vi "Decimate 1D by Min-Max Algorythm.vi"(4 "Width":i32, 6 "Packet sizes":i32[](array[numeric]), 8 "error in (no error)":errorcluster, 9 "Min Index":i32, 10 "Max Index":i32, 11 "Data To Decimate":dbl[](array[numeric])) -> (0 "error out":errorcluster, 3 "Decimated Data":dbl[](array[numeric]))   [LabVIEW 2022 SP3, in "Decimation.lvlib"]
uses:
  Decimation.lvlib
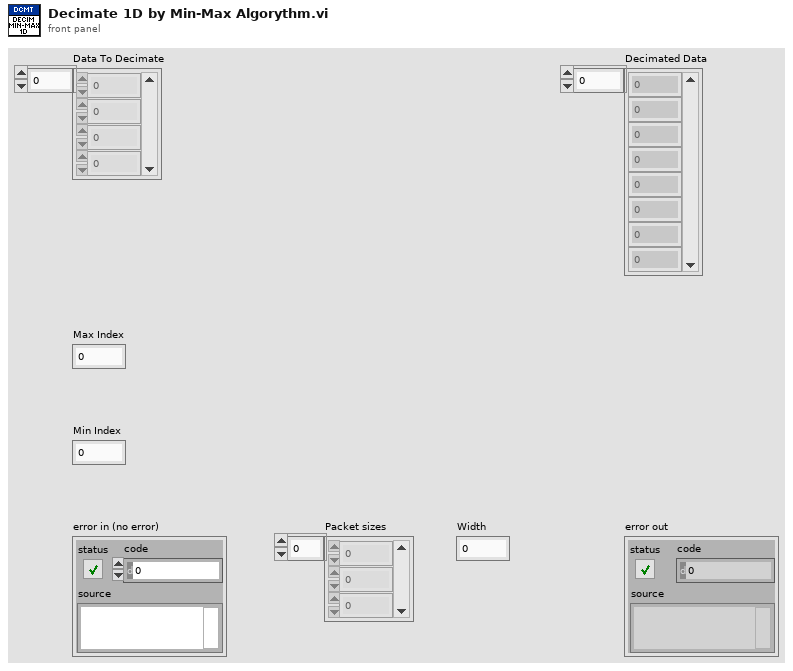
[diagram p1: front panel]
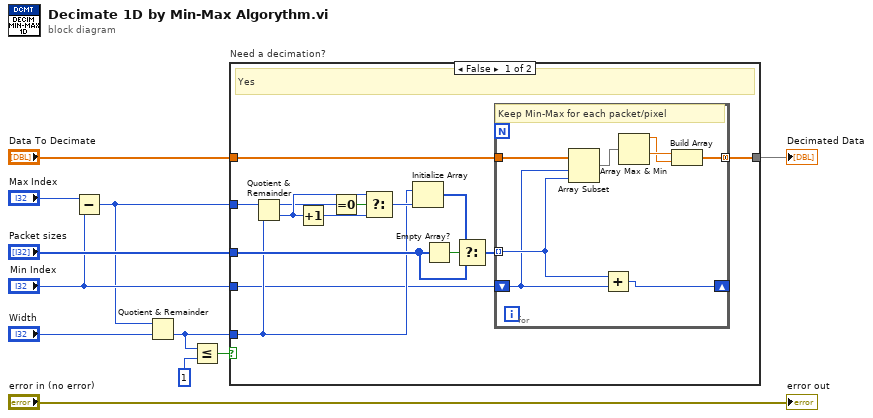
[diagram p0: block diagram]
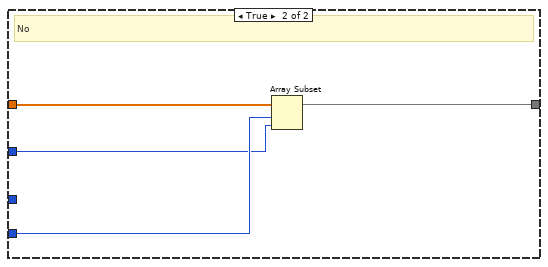
[diagram p2: hidden frame]
diagram:
  n1 = Subtract(x="Max Index", y="Min Index") -> (x-y=w1:i32)
  n2 = Quotient & Remainder(x=w1, y="Width") -> (floor(x/y)=w2:i32)  [unwired: 1 out]
  n3 = Less Or Equal?(x=w2, y=u32 1) -> (x <= y?=w6:bool)
  n4 = case "Need a decimation?" shown="False" w6 {
    tunnel: "Packet sizes" -> [w22 _]
    tunnel: "Data To Decimate" -> [w25 w37]
    tunnel: [w24 w36] -> w11
    tunnel: "Min Index" -> [w12 w35]
    tunnel: w2 -> [w13 _]
    tunnel: w1 -> [w20 w34]
    frame False {
      # "Yes"
      n5 = Quotient & Remainder(x=w20, y=w13) -> (x-y*floor(x/y)=w16:i32, floor(x/y)=w17:i32)
      n6 = Increment(x=w17) -> (x+1=w18:i32)
      n7 = Equal To 0?(x=w16) -> (x = 0?=w19:bool)
      n8 = Select(t=w17, s=w19, f=w18) -> (s? t:f=w14:i32)
      n9 = Initialize Array(w13, w14) -> (w15:i32[])
      n10 = Empty Array?(array=w22) -> (empty?=w23:bool)
      n11 = Select(t=w15, s=w23, f=w22) -> (s? t:f=w21:i32[])
      n12 = for {
        tunnel: [w32] -> w24 mode=concatenating
        tunnel: w21 -> [w28] mode=indexing
        shift-right: [w26] -> _
        shift-left: w12 -> [w27]
        tunnel: w25 -> [w33]
        # "Keep Min-Max for each packet/pixel"
        n13 = Array Subset(array=w33, index=w27, length=w28) -> (w31:dbl[])
        n14 = Add(x=w28, y=w27) -> (x+y=w26:i32)
        n15 = Array Max & Min(array=w31) -> (max value=w29:dbl, min value=w30:dbl)  [unwired: 2 out]
        n16 = Build Array(w30, w29) -> (w32:dbl[])
      }
    }
    frame True {
      # "No"
      n17 = Array Subset(array=w37, index=w35, length=w34) -> (w36:dbl[])
    }
  }
  "Decimated Data" <- w11
  "error out" <- "error in (no error)"
